vi "FVIR_Alicat_GasMeter.vi"(8 "error in":errorcluster, 10 "VISA Refnum in":refnum<visa-resource-name>="ALICAT_100SLPM", 11 "Message Queues":T2) -> (0 "error out":errorcluster)   [LabVIEW 2020]
uses:
  Message Queue/All Message Queues.ctl
  Message Queue/Message Cluster.ctl
  Drivers/Alicat LabVIEW Drivers 2v1/Sub-VIs/Data Cluster.ctl
  Modbus/Modbus Gas Meter Data.ctl
  Drivers/Alicat LabVIEW Drivers 2v1/Sub-VIs/Units of Measure.ctl
  Message Queue/Enqueue Message (Single).vi
  Message Queue/Message Queue.lvlib
panel:
  out "Data Cluster":T1
  in  "Trigger Error?":bool
  in  "Debug":bool
  out "Debug":string[](array[string])
  # "Totalizer Timer"
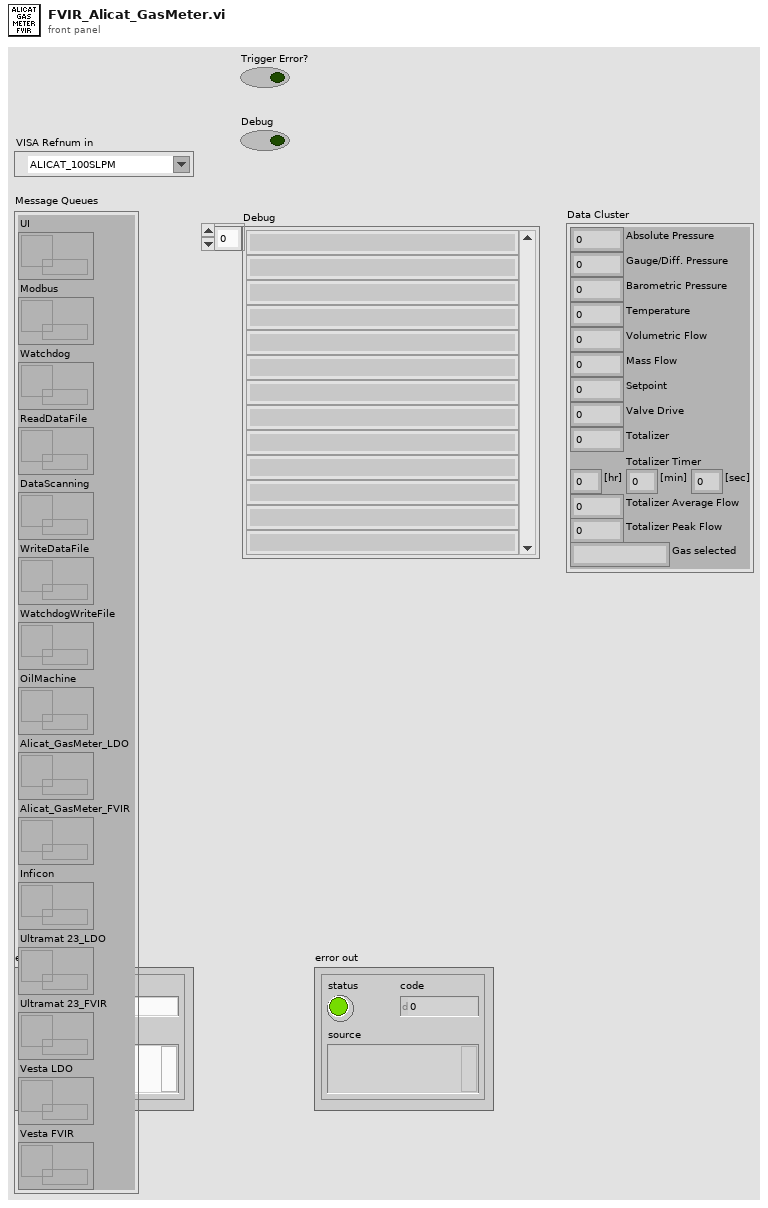
[diagram p1: front panel]
types:
  T1 = typedef "Data Cluster.ctl" = cluster{"Absolute Pressure":dbl, "Gauge/Diff. Pressure":dbl, "Barometric Pressure":dbl, "Temperature":dbl, "Volumetric Flow":dbl, "Mass Flow":dbl, "Setpoint":dbl, "Valve Drive":dbl, "Totalizer":dbl, "[hr]":dbl, "[min]":dbl, "[sec]":dbl, "Totalizer Average Flow":dbl, "Totalizer Peak Flow":dbl, "Gas selected":string}
  T2 = typedef "Message Queue.lvlib/All Message Queues.ctl" = cluster{"UI":refnum<queue>, "Modbus":refnum<queue>, "Watchdog":refnum<queue>, "ReadDataFile":refnum<queue>, "DataScanning":refnum<queue>, "WriteDataFile":refnum<queue>, "WatchdogWriteFile":refnum<queue>, "OilMachine":refnum<queue>, "Alicat_GasMeter_LDO":refnum<queue>, "Inficon":refnum<queue>, "Ultramat 23_LDO":refnum<queue>, "Alicat_GasMeter_FVIR":refnum<queue>, "Ultramat 23_FVIR":refnum<queue>, "Vesta LDO":refnum<queue>, "Vesta FVIR":refnum<queue>}
  T3 = cluster{"Absolute Press.":bool, "Gauge/Diff. Press.":bool, "Barometric Press.":bool, "Temperature":bool, "Volumetric":bool, "Mass Flow":bool, "Setpoint":bool, "Valve Drive":bool, "Totalizer":bool, "Tot. Timer [s]":bool, "Tot. Avg. Flow":bool, "Tot. Peak Flow":bool, "Gas Selected":bool, "Log Data":bool}
  T4 = typedef "Modbus Gas Meter Data.ctl" = cluster{"Data Cluster":T1, "Units of Measure Input":T5, "Header Array":string[]}
  T5 = typedef "Units of Measure.ctl" = cluster{"Abs. Pressure":string, "Gauge/Diff. Press.":string, "Barometric Press.":string, "Temperature":string, "Volume":string, "Mass":string, "Setpoint":string, "Valve Drive":string, "Totalizer":string, "Tot. Timer":string, "Tot. Avg. Flow":string, "Tot. Peak Flow":string}
  T6 = typedef "Data Frame.ctl" = cluster{"Absolute Pressure":bool, "Gauge/Diff. Pressure":bool, "Barometric Pressure":bool, "Temperature":bool, "Volumetric":bool, "Mass":bool, "Setpoint":bool, "Valve Drive":bool, "Totalizer":bool, "Totalizer Timer":bool, "Totalizer Average Flow":bool, "Totalizer Peak Flow":bool, "Gas Selected":bool, "Tot. Timer Format":u16}
  T7 = typedef "FMA1600A Units String.ctl" = cluster{"Software Rev":string, "Model Number":string, "Manufacturer Info":string, "Software Sub-Rev":string, "Board Rev":string, "Units of Measure Input":T5}
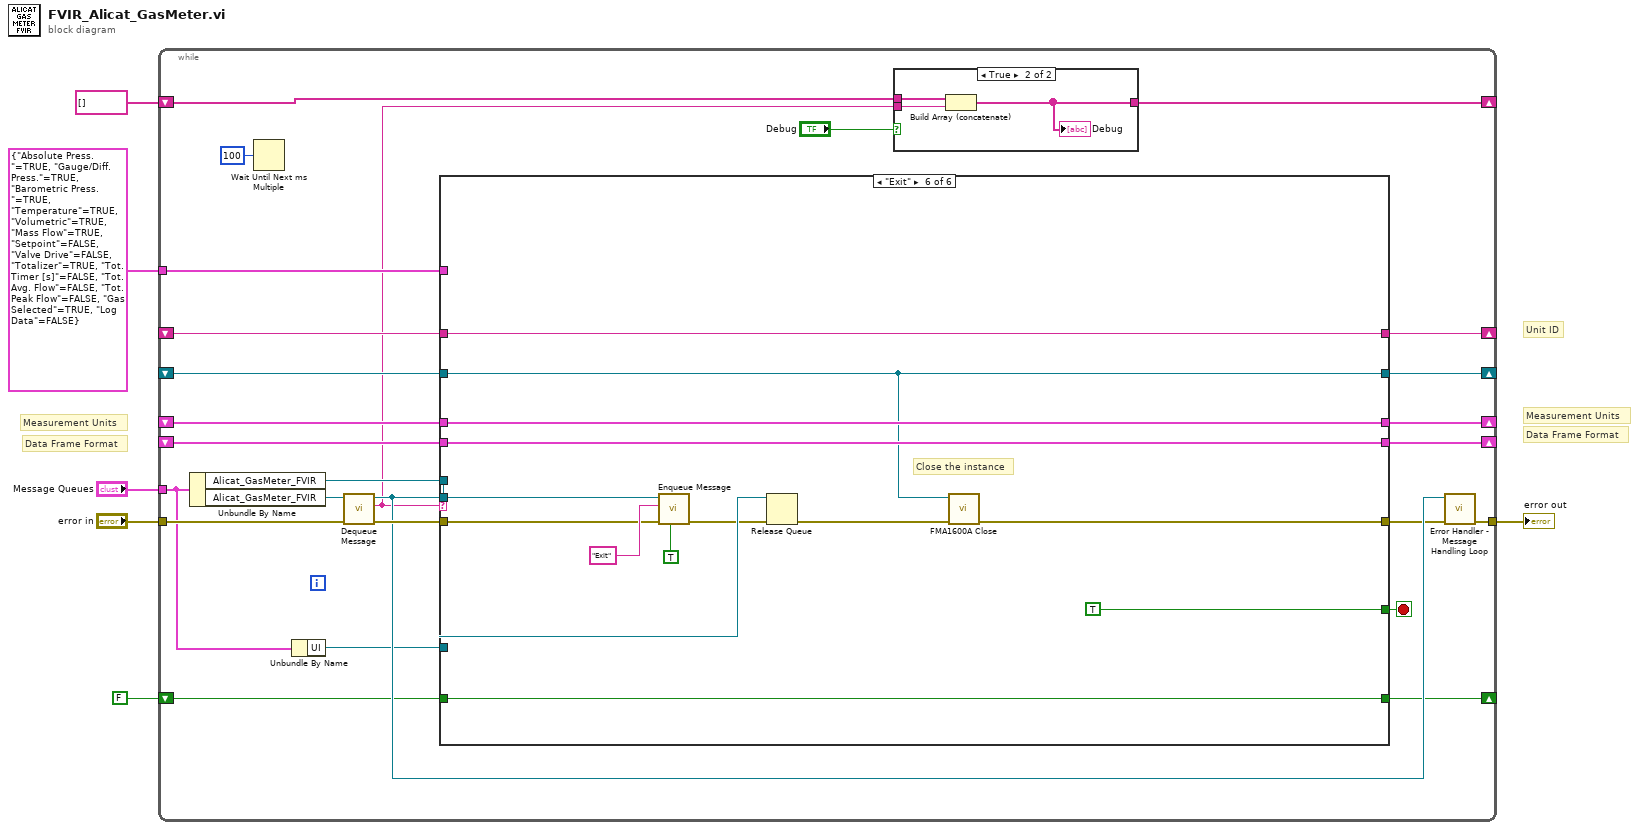
[diagram p0: block diagram]
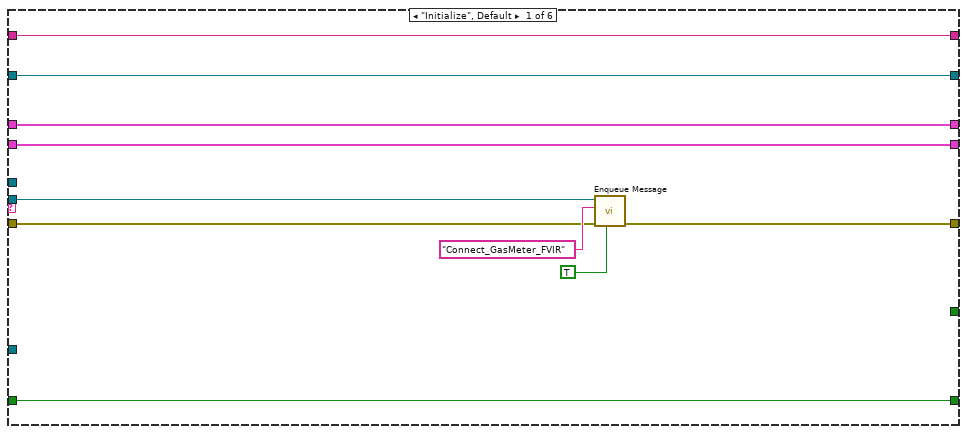
[diagram p3: hidden frame]
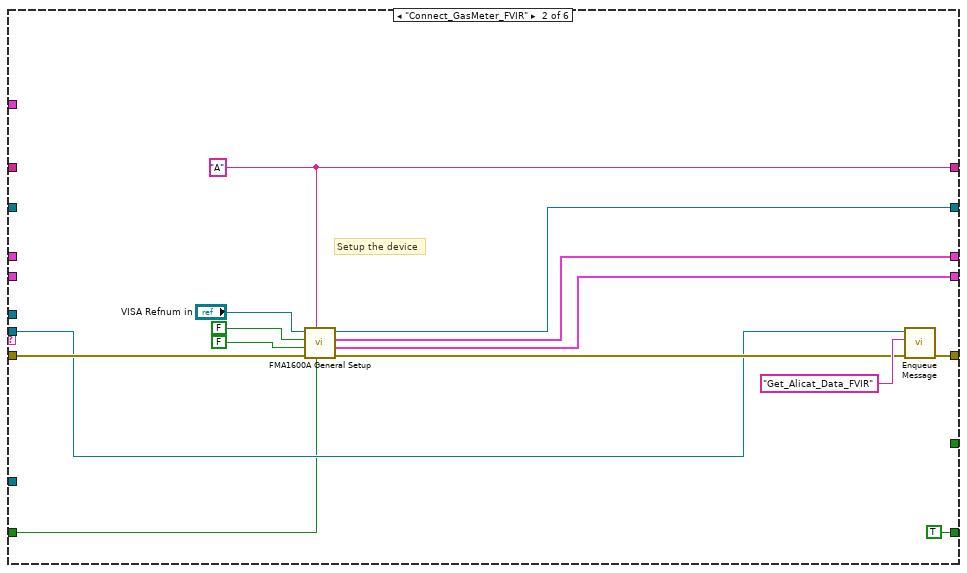
[diagram p4: hidden frame]
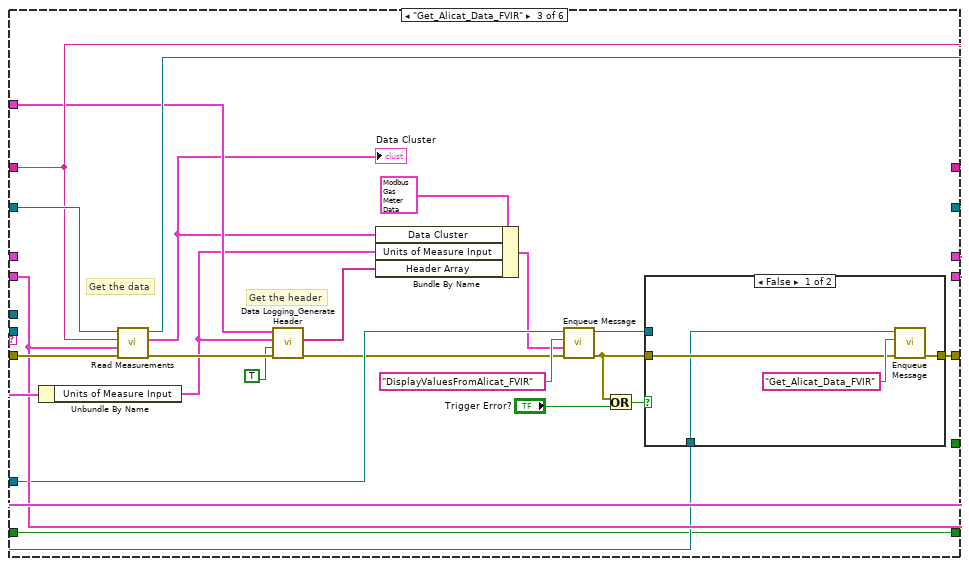
[diagram p5: hidden frame]
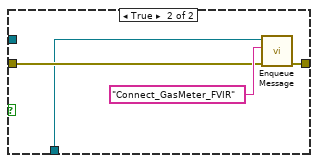
[diagram p6: hidden frame]
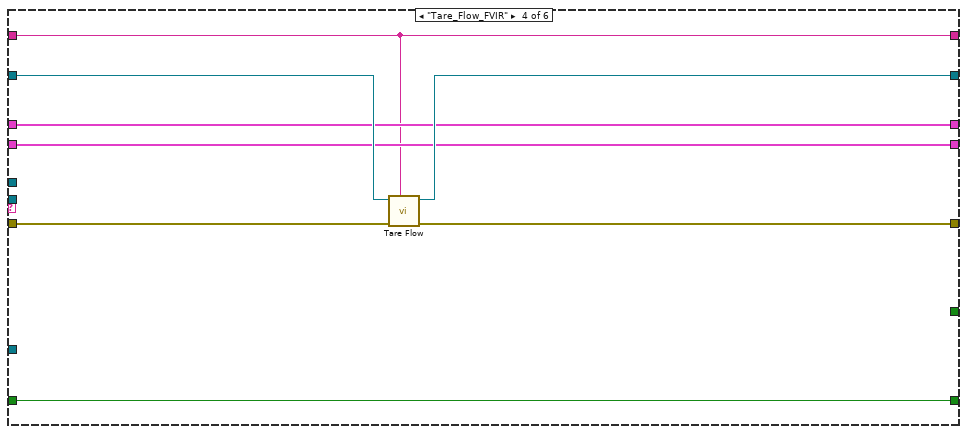
[diagram p7: hidden frame]
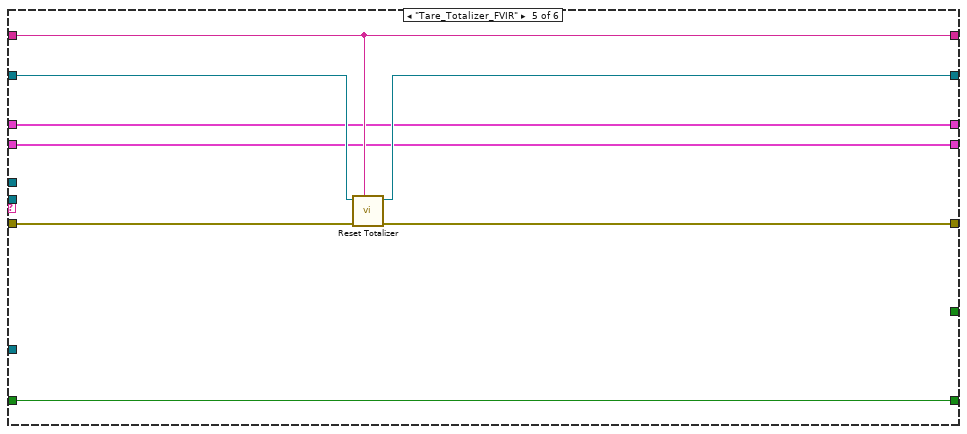
[diagram p8: hidden frame]
diagram:
  # "Unit ID"
  # "Data Frame Format"
  # "Measurement Units"
  # "Unit ID"
  # "Data Frame Format"
  # "Measurement Units"
  n1 = while {
    tunnel: "Message Queues" -> [w14]
    tunnel: "error in" -> [w31]
    tunnel: [w26] -> w4
    shift-right: [w24] -> _
    shift-left: _ -> [w23]
    shift-right: [w21] -> _
    shift-left: _ -> [w18]
    shift-right: [w20] -> _
    shift-left: _ -> [w19]
    shift-right: [w17] -> _
    shift-left: _ -> [w16]
    tunnel: T3 {"Absolute Press."=TRUE, "Gauge/Diff. Press."=TRUE, "Barometric Press."=TRUE, "Temperature"=TRUE, "Volumetric"=TRUE, "Mass Flow"=TRUE, "Setpoint"=FALSE, "Valve Drive"=FALSE, "Totalizer"=TRUE, "Tot. Timer [s]"=FALSE, "Tot. Avg. Flow"=FALSE, "Tot. Peak Flow"=FALSE, "Gas Selected"=TRUE, "Log Data"=FALSE} ("Data Logging Options") -> [w15]
    shift-right: [w10] -> _
    shift-left: string[] [] -> [w11]
    shift-right: [w7] -> _
    shift-left: FALSE -> [w8]
    stop <- w29 stop-if-true
    n2 = Unbundle By Name(w14) -> ("Alicat_GasMeter_FVIR"=w28:refnum<queue>, "Alicat_GasMeter_FVIR"=w32:refnum<queue>)
    n3 = Wait Until Next ms Multiple(millisecond multiple=u32 100) -> ()  [unwired: 1 out]
    n4 = Unbundle By Name(w14) -> ("UI"=w13:refnum<queue>)
    n5 = call "Dequeue Message.vi"("error in (no error)"=w31, "Message Queue"=w32) -> ("error out"=w30:errorcluster, "Message"=w12:string, "dup Message Queue"=w27:refnum<queue>)  [unwired: 6 in, 1 out]
    n6 = case shown="\"Exit\"" w12 {
      tunnel: w30 -> [w41 w57 w81 w100 w108 w118]
      tunnel: [w40 w51 w73 w99 w107 w114] -> w25
      tunnel: [_ _ _ _ _ TRUE] -> w29
      tunnel: w28 -> [_ _ _ _ _ w119]
      tunnel: w27 -> [w39 w50 w72 _ _ w117]
      tunnel: [w46 w56 w82 w97 w104 w110] -> w24
      tunnel: w23 -> [w46 _ w80 w98 w106 w110]
      tunnel: [w44 w55 w78 w96 w103 w112] -> w21
      tunnel: [w43 w54 w77 w95 w102 w111] -> w20
      tunnel: w19 -> [w43 _ w77 w95 w102 w111]
      tunnel: w18 -> [w44 _ w78 w96 w103 w112]
      tunnel: [w45 w49 w79 w94 w105 w113] -> w17
      tunnel: w16 -> [w45 _ w79 w94 w105 w113]
      tunnel: w15 -> [_ _ w76 _ _ _]
      tunnel: w13 -> [_ _ w74 _ _ _]
      tunnel: w8 -> [w37 w48 w61 w93 w101 w109]
      tunnel: [w37 TRUE w61 w93 w101 w109] -> w7
      frame "Initialize", Default {
        n7 = call-poly "Enqueue Message.vi"("Priority Message? (F)"=TRUE, "error in (no error)"=w41, "Message"="Connect_GasMeter_FVIR", "Message Queue"=w39) -> ("error out"=w40:errorcluster)  [unwired: 6 in, 1 out]
      }
      frame "Connect_GasMeter_FVIR" {
        w49 = "A" ("Unit ID")
        # "Setup the device"
        n8 = call "FMA1600A General Setup.vi"("Skip Dialog"=w48, "Unit ID"=w49, "error in (no error)"=w57, "Select Gas?"=FALSE, "Set STP Register"=FALSE, "VISA Refnum in"="VISA Refnum in") -> ("error out"=w52:errorcluster, "Data Frame Format"=w54:T6, "Measurement Units"=w55:T7, "VISA Refnum out"=w56:refnum<visa-resource-name>)  [unwired: 2 in]
        n9 = call-poly "Enqueue Message.vi"("error in (no error)"=w52, "Message"="Get_Alicat_Data_FVIR", "Message Queue"=w50) -> ("error out"=w51:errorcluster)  [unwired: 7 in, 1 out]
      }
      frame "Get_Alicat_Data_FVIR" {
        # "Get the header"
        # "Get the data"
        n10 = Unbundle By Name(w78) -> ("Units of Measure Input"=w68:T5)
        n11 = call "Read Measurements.vi"("error in"=w81, "Data Frame Format In"=w77, "Unit ID (A)"=w79, "VISA Session In"=w80) -> ("error out"=w84:errorcluster, "Data Cluster"=w69:T1, "VISA Session Out"=w82:refnum<visa-resource-name>)  [unwired: 5 out]
        "Data Cluster" <- w69
        n12 = call "Data Logging_Generate Header.vi"("error in"=w84, "Include Units\nin Header (F)"=TRUE ("Include Units\nin Header (default is F)"), "Units of Measure Input"=w68, "Data Logging Options"=w76) -> ("error out"=w71:errorcluster, "Header Array"=w67:string[])  [unwired: 5 in, 1 out]
        n13 = Bundle By Name(cluster=T4 {"Data Cluster"={"Absolute Pressure"=0.0, "Gauge/Diff. Pressure"=0.0, "Barometric Pressure"=0.0, "Temperature"=0.0, "Volumetric Flow"=0.0, "Mass Flow"=0.0, "Setpoint"=0.0, "Valve Drive"=0.0, "Totalizer"=0.0, "[hr]"=0.0, "[min]"=0.0, "[sec]"=0.0, "Totalizer Average Flow"=0.0, "Totalizer Peak Flow"=0.0, "Gas selected"=""}, "Units of Measure Input"={"Abs. Pressure"="", "Gauge/Diff. Press."="", "Barometric Press."="", "Temperature"="", "Volume"="", "Mass"="", "Setpoint"="", "Valve Drive"="", "Totalizer"="", "Tot. Timer"="", "Tot. Avg. Flow"="", "Tot. Peak Flow"=""}, "Header Array"=[]} ("Gas Data"), "Data Cluster"=w69, "Units of Measure Input"=w68, "Header Array"=w67) -> (w66:T4)
        n14 = call-poly "Enqueue Message.vi"("error in (no error)"=w71, "Message Data"=w66, "Message"="DisplayValuesFromAlicat_FVIR", "Message Queue"=w74) -> ("error out"=w64:errorcluster, "dup Message Queue"=w65:refnum<queue>)  [unwired: 6 in]
        n15 = Or(x=w64, y="Trigger Error?") -> (x .or. y?=w63:bool)
        n16 = case shown="False" w63 {
          tunnel: w64 -> [w87 w90]
          tunnel: [w86 w91] -> w73
          tunnel: w72 -> [w85 w89]
          tunnel: w65 -> [_ _]
          frame False {
            n17 = call-poly "Enqueue Message.vi"("error in (no error)"=w87, "Message"="Get_Alicat_Data_FVIR", "Message Queue"=w85) -> ("error out"=w86:errorcluster)  [unwired: 7 in, 1 out]
          }
          frame True {
            n18 = call-poly "Enqueue Message.vi"("error in (no error)"=w90, "Message"="Connect_GasMeter_FVIR", "Message Queue"=w89) -> ("error out"=w91:errorcluster)  [unwired: 7 in, 1 out]
          }
        }
      }
      frame "Tare_Flow_FVIR" {
        n19 = call "Tare Flow.vi"("Unit ID (A)"=w94, "error in"=w100, "VISA Session In"=w98) -> ("error out"=w99:errorcluster, "VISA Session Out"=w97:refnum<visa-resource-name>)  [unwired: 7 in]
      }
      frame "Tare_Totalizer_FVIR" {
        n20 = call "Reset Totalizer.vi"("Unit ID (A)"=w105, "error in"=w108, "VISA Session In"=w106) -> ("error out"=w107:errorcluster, "VISA Session Out"=w104:refnum<visa-resource-name>)  [unwired: 6 in, 1 out]
      }
      frame "Exit" {
        # "Close the instance"
        n21 = call-poly "Enqueue Message.vi"("Priority Message? (F)"=TRUE, "error in (no error)"=w118, "Message"="Exit", "Message Queue"=w119) -> ("error out"=w116:errorcluster)  [unwired: 6 in, 1 out]
        n22 = Release Queue(queue=w117, error in (no error)=w116) -> (error out=w115:errorcluster)  [unwired: 1 in, 2 out]
        n23 = call "FMA1600A Close.vi"("error in (no error)"=w115, "VISA Refnum in"=w110) -> ("error out"=w114:errorcluster)  [unwired: 9 in]
      }
    }
    n24 = case shown="True" "Debug" {
      tunnel: w12 -> [_ w36]
      tunnel: w11 -> [w33 w35]
      tunnel: [w33 w34] -> w10
      frame False {
      }
      frame True {
        n25 = Build Array (concatenate)(w35, w36) -> (w34:string[])
        "Debug" <- w34
      }
    }
    n26 = call "Error Handler - Message Handling Loop.vi"("error in (no error)"=w25, "Message Queue"=w27) -> ("dup error in"=w26:errorcluster)  [unwired: 8 in, 1 out]
  }
  "error out" <- w4
